vi "Untitled 4.vi"() -> ()   [LabVIEW 2016, in "Logger.syslog.lvclass"]
uses:
  Logger.syslog.lvclass
  <userlib>/_MGI/Error Reporter/MGI Error Reporter Dialog/MGI Error Reporter Dialog.lvclass
  C:/Program Files (x86)/National Instruments/LabVIEW 2016/user.lib/_MGI/Error Reporter/MGI Error Reporter Base/MGI Error Reporter Base.lvclass
  <userlib>/_OpenG.lib/numeric/numeric.llb/Random Number Within Range - DBL__ogtk.vi
  <userlib>/_MGI/Error Reporter/MGI Error Reporter Base/MGI Error Reporter Base.lvclass
panel:
  out "Already Running?":bool
  out "Error Log Directory Used":path
  in  "Log Error":bool
  in  "Stop":bool
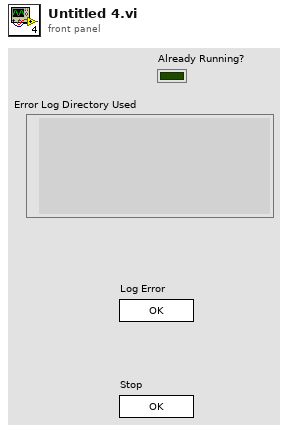
[diagram p1: front panel]
types:
  T1 = enum32{"Invalid", "Standard", "Closed", "Hidden", "Minimized", "Maximized"}
  T2 = enum32{"invalid app kind", "Development System", "Run Time System", "Student Edition", "Embedded LabVIEW", "Evaluation", "Custom"}
  T3 = cluster{"Core":cluster{"Current VI Reference":refnum<vi>, "Close Panel on Exit?":bool}, "Your Boolean data":bool, "Your string data":string}
  T4 = cluster{"Current VI Reference":refnum<vi>, "Close Panel on Exit?":bool}
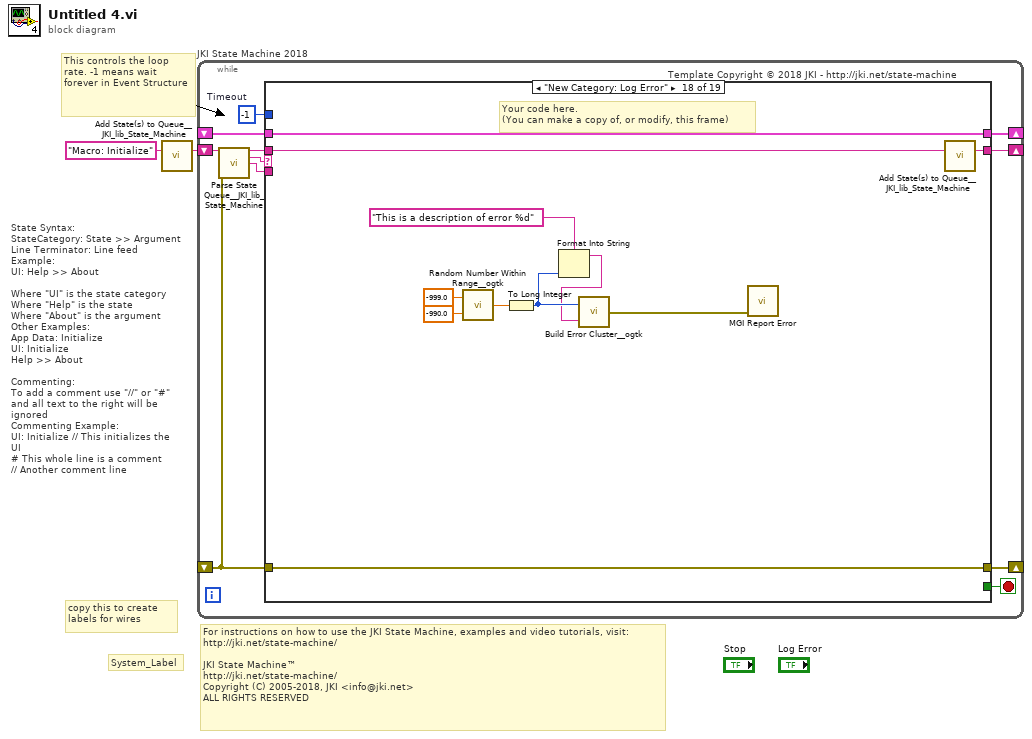
[diagram p0: block diagram]
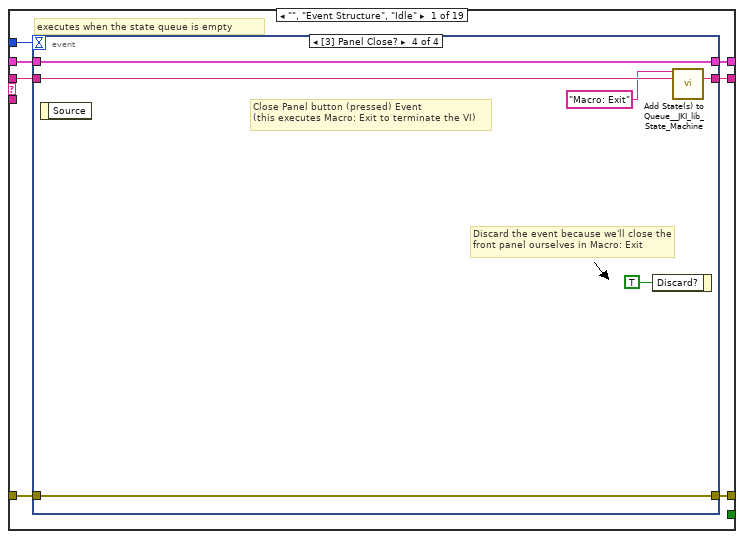
[diagram p2: hidden frame]
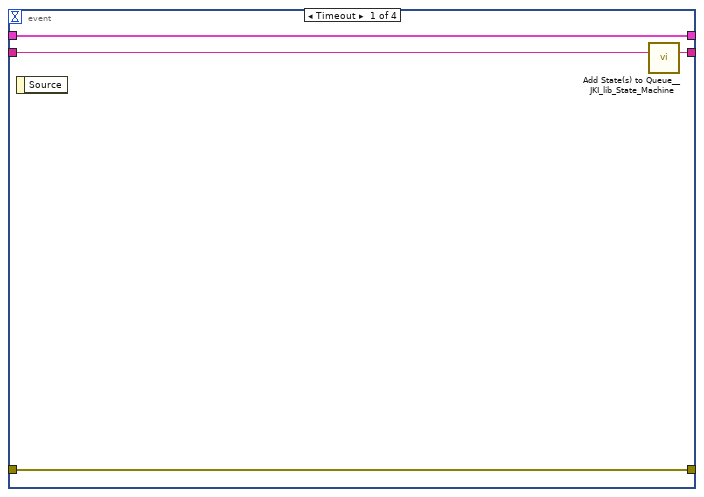
[diagram p3: hidden frame]
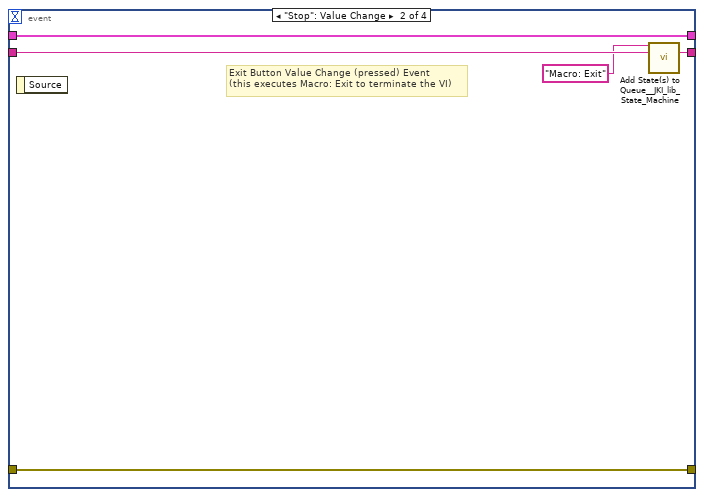
[diagram p4: hidden frame]
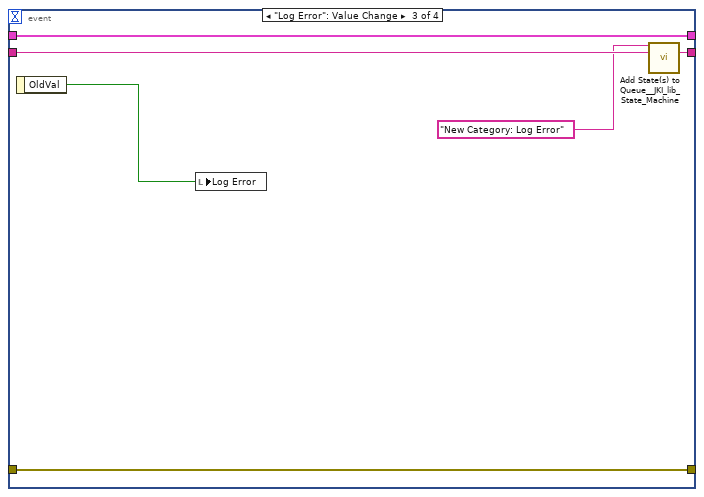
[diagram p5: hidden frame]
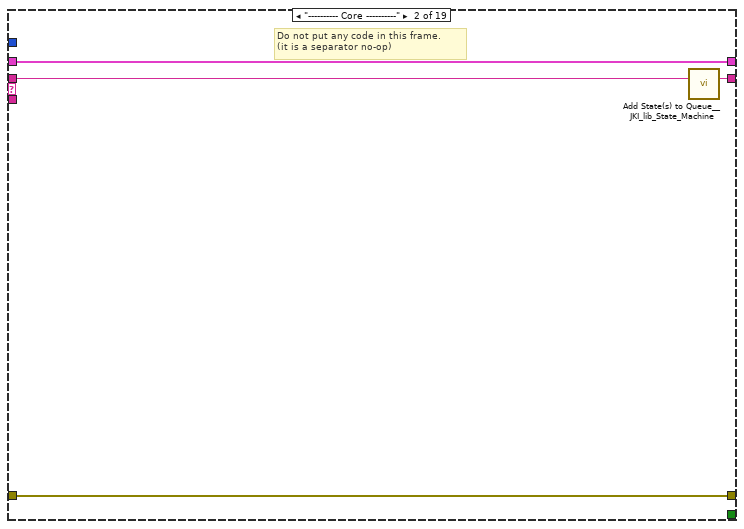
[diagram p6: hidden frame]
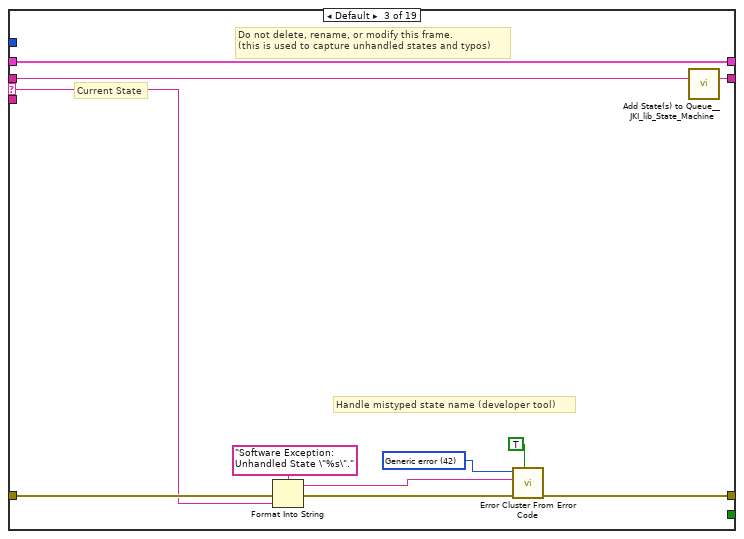
[diagram p7: hidden frame]
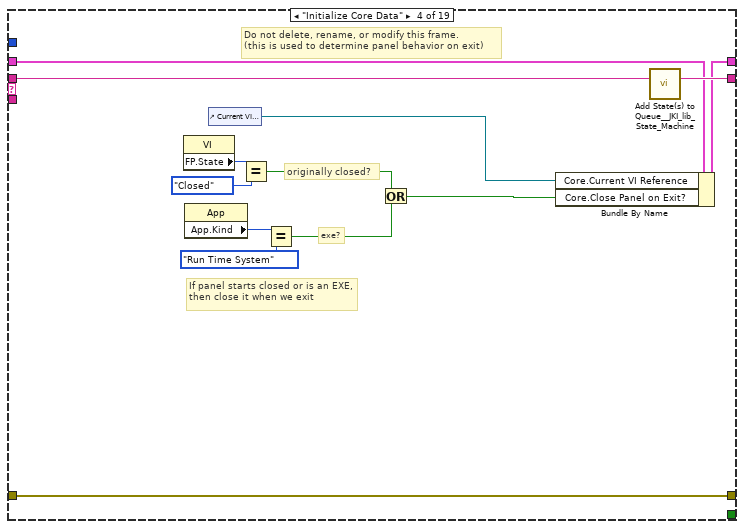
[diagram p8: hidden frame]
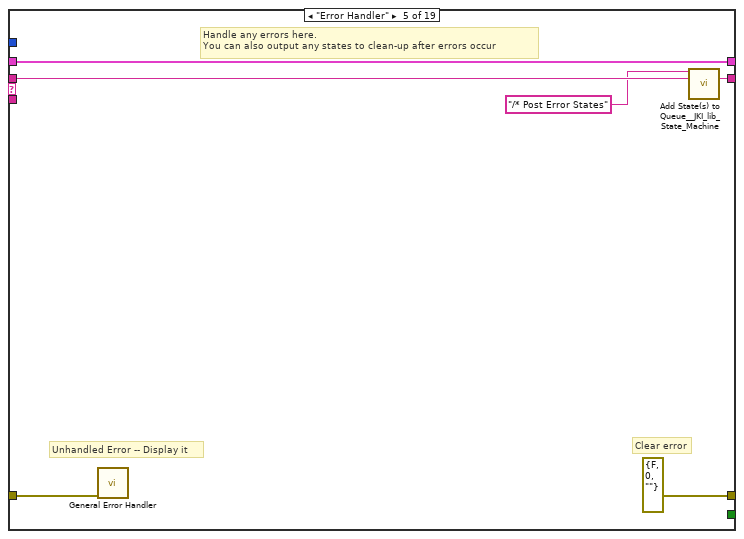
[diagram p9: hidden frame]
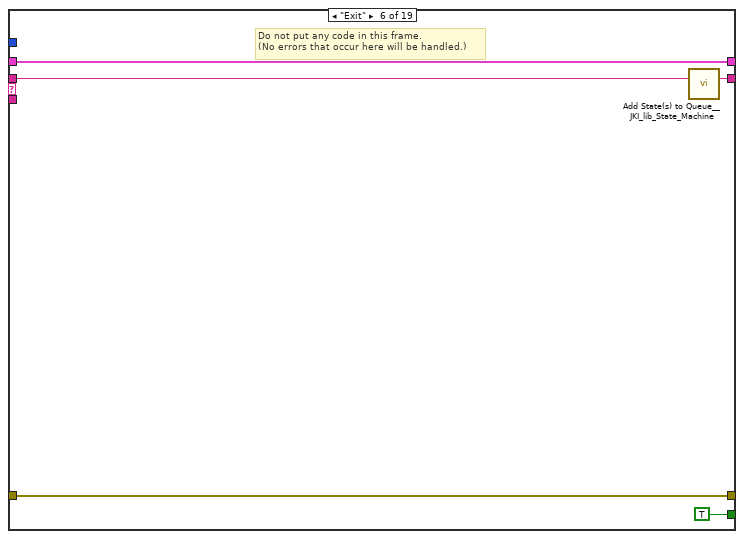
[diagram p10: hidden frame]
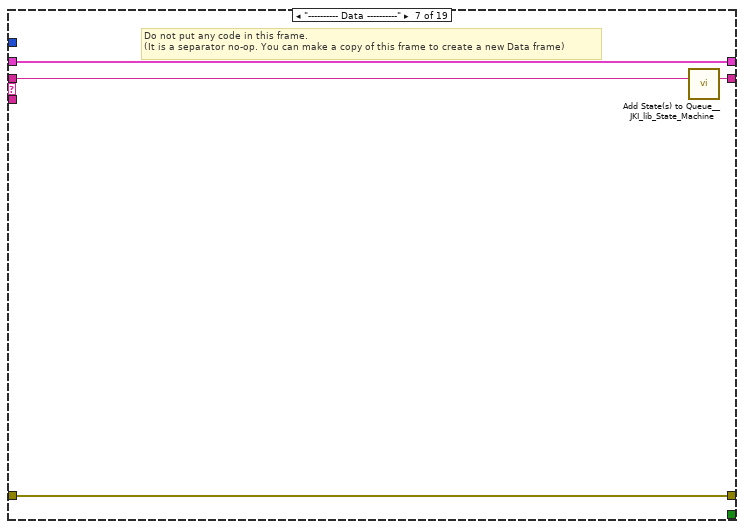
[diagram p11: hidden frame]
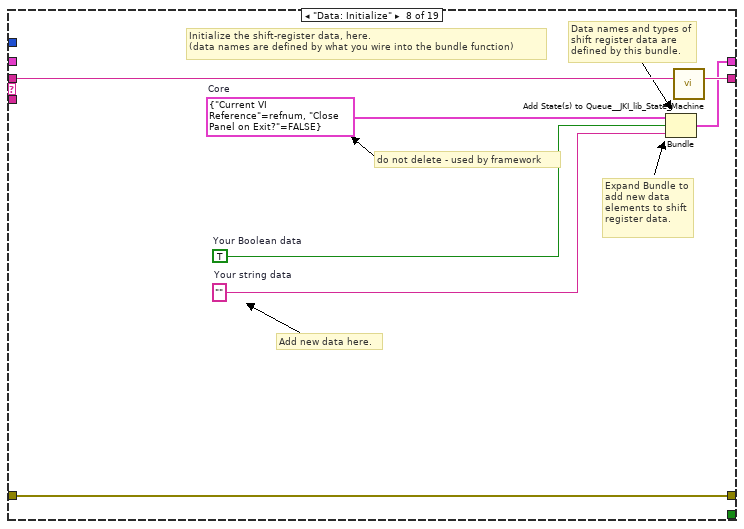
[diagram p12: hidden frame]
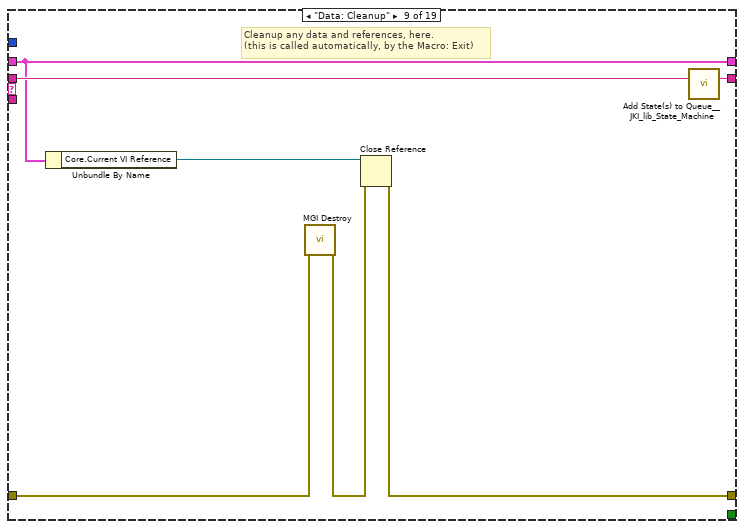
[diagram p13: hidden frame]
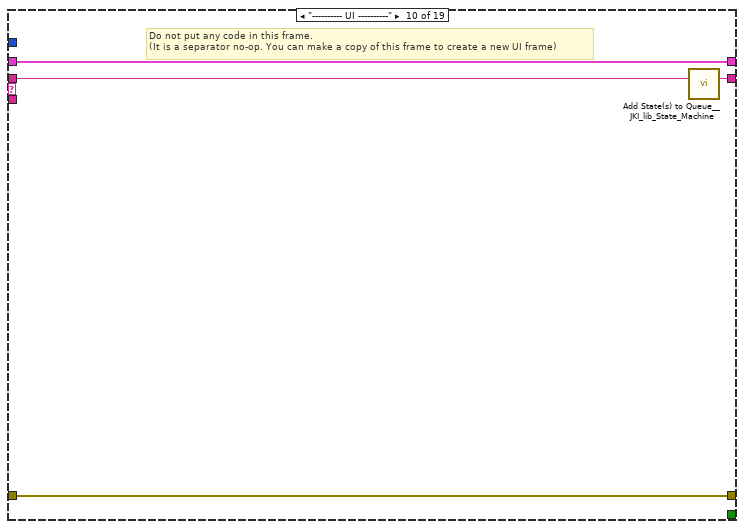
[diagram p14: hidden frame]
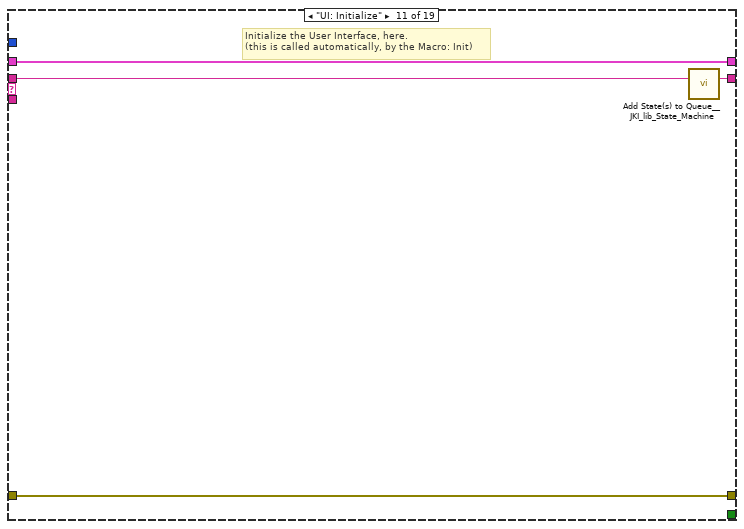
[diagram p15: hidden frame]
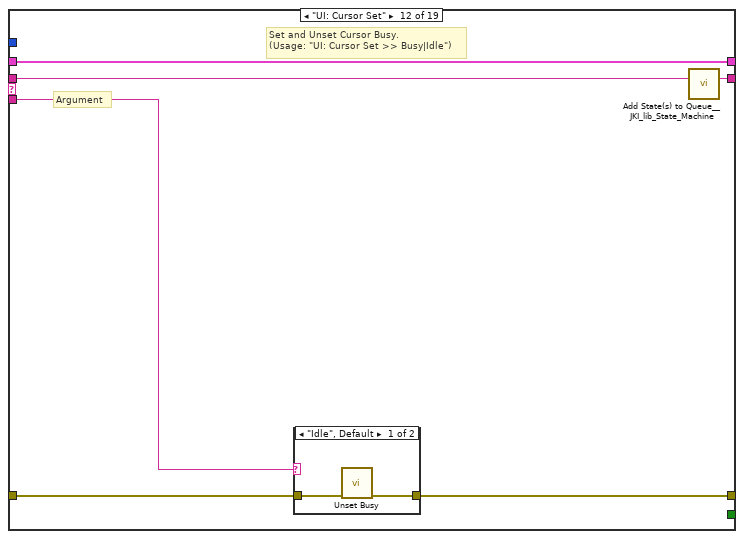
[diagram p16: hidden frame]
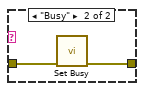
[diagram p17: hidden frame]
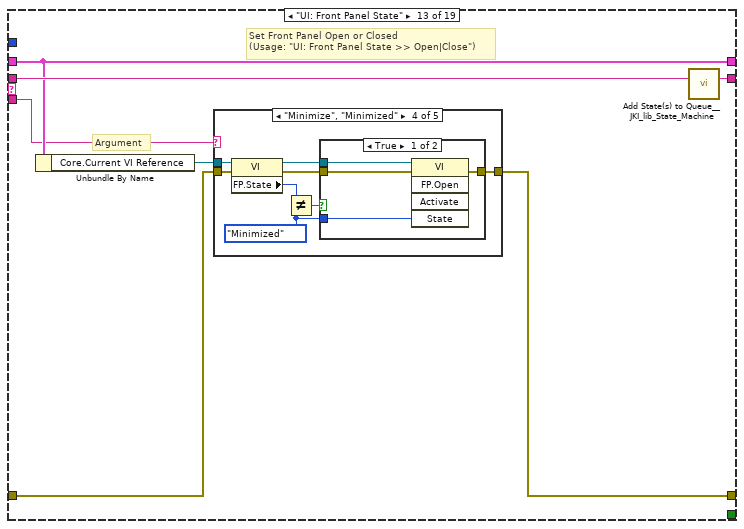
[diagram p18: hidden frame]
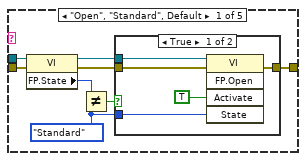
[diagram p19: hidden frame]
diagram:
  # "For instructions on how to use the JKI State Machine, examples and video tutorials, visit:\nhttp://jki.net/state-machine/\n\nJKI State Machine™\nhttp://jki.net/state-machine/\nCopyright (C) 2005-2018, JKI <info@jki.net>\nALL RIGHTS RESERVED"
  # "State Syntax:\nStateCategory: State >> Argument\nLine Terminator: Line feed\nExample:\nUI: Help >> About\n\nWhere \"UI\" is the state category\nWhere \"Help\" is the state\nWhere \"About\" is the argument\nOther Examples:\nApp Data: Initialize\nUI: Initialize\nHelp >> About\n\nCommenting:\nTo add a comment use \"//\" or \"#\" and all text to the right will be ignored\nCommenting Example:\nUI: Initialize // This initializes the UI\n# This whole line is a comment\n// Another comment line"
  # "copy this to create labels for wires"
  # "This controls the loop rate. -1 means wait forever in Event Structure"
  # "System_Label"
  n1 = call <vilib>:"Add State(s) to Queue__JKI_lib_State_Machine.vi"("State(s) in (\"\")"="Macro: Initialize") -> ("States Out"=w2:string)  [unwired: 14 in]
  n2 = while "JKI State Machine 2018" {
    shift-right: [w6] -> _
    shift-left: _ -> [w5]
    shift-right: [w9] -> _
    shift-left: _ -> [w3]
    shift-right: [w8] -> _
    shift-left: w2 -> [w10]
    stop <- w7 stop-if-true
    w4 = -1  # Timeout
    # "Template Copyright © 2018 JKI - http://jki.net/state-machine"
    n3 = call <vilib>:"Parse State Queue__JKI_lib_State_Machine.vi"("State Queue"=w10, "Error In (no error)"=w3) -> ("Remaining States"=w12:string, "Current State"=w13:string, "Arguments"=w11:string)  [unwired: 11 in]
    n4 = case shown="\"New Category: Log Error\"" w13 {
      selector: w13 -> [_ _ w46 _ _ _ _ _ _ _ _ _ _ _ _ _ _ _ _]
      tunnel: w12 -> [w20 w45 w50 w69 w75 w80 w84 w91 w98 w102 w106 w112 w123 w192 w197 w207 w211 w222 w240]
      tunnel: w11 -> [_ _ _ _ _ _ _ _ _ _ _ w107 w117 _ _ _ _ _ _]
      tunnel: w5 -> [w18 w42 w48 w62 w72 w78 w81 _ w94 w99 w104 w110 w119 w189 w194 w204 w208 w220 w238]
      tunnel: [w17 w43 w52 w66 errorcluster {"status"=FALSE, "code"=0, "source"=""} ("error out") w77 w82 w88 w95 w100 w103 w108 w120 w190 w195 w205 w209 w216 w235] -> w9
      tunnel: w3 -> [w16 w43 w51 w66 w71 w77 w82 w88 w93 w100 w103 w109 w121 w190 w195 w205 w209 w216 w236]
      tunnel: [w19 w44 w49 w68 w74 w79 w83 w90 w97 w101 w105 w111 w122 w191 w196 w206 w210 w221 w239] -> w8
      tunnel: [_ _ _ _ _ TRUE _ _ _ _ _ _ _ _ _ _ _ _ _] -> w7
      tunnel: [w15 w42 w48 w67 w72 w78 w81 w89 w94 w99 w104 w110 w119 w189 w194 w204 w208 w220 w238] -> w6
      tunnel: w4 -> [w14 _ _ _ _ _ _ _ _ _ _ _ _ _ _ _ _ _ _]
      frame "", "Event Structure", "Idle" {
        # "executes when the state queue is empty"
        n5 = event shown="[3] Panel Close?" {
          selector: _ -> [_ _ _ _]
          dyn-events: _ -> [_ _ _ _]
          timeout: w14 -> [_ _ _ _]
          tunnel: w20 -> [w24 w29 w35 w41]
          tunnel: [w23 w28 w34 w40] -> w19
          tunnel: w18 -> [w21 w26 w32 w38]
          tunnel: [w22 w27 w33 w39] -> w17
          tunnel: w16 -> [w22 w27 w33 w39]
          tunnel: [w21 w26 w32 w38] -> w15
          event Timeout {
            n6 = event-data() -> ()  [unwired: 1 in, 1 out]
            n7 = call <vilib>:"Add State(s) to Queue__JKI_lib_State_Machine.vi"("State(s) in (\"\")"=w24) -> ("States Out"=w23:string)  [unwired: 14 in]
          }
          event "Stop": Value Change {
            # "Exit Button Value Change (pressed) Event\n(this executes Macro: Exit to terminate the VI)"
            n8 = event-data() -> ()  [unwired: 1 in, 1 out]
            n9 = call <vilib>:"Add State(s) to Queue__JKI_lib_State_Machine.vi"("State(s) in Front (\"\")"="Macro: Exit", "State(s) in (\"\")"=w29) -> ("States Out"=w28:string)  [unwired: 13 in]
          }
          event "Log Error": Value Change {
            n10 = event-data() -> ("OldVal"=w30:bool)  [unwired: 1 in]
            n11 = local write "Log Error"(w30) -> ()
            n12 = call <vilib>:"Add State(s) to Queue__JKI_lib_State_Machine.vi"("State(s) in Front (\"\")"="New Category: Log Error", "State(s) in (\"\")"=w35) -> ("States Out"=w34:string)  [unwired: 13 in]
          }
          event Panel Close? {
            # "Discard the event because we'll close the front panel ourselves in Macro: Exit"
            # "Close Panel button (pressed) Event\n(this executes Macro: Exit to terminate the VI)"
            n13 = event-data() -> ()  [unwired: 1 in, 1 out]
            n14 = event-data("Discard?"=TRUE) -> ()  [unwired: 1 in, 1 out]
            n15 = call <vilib>:"Add State(s) to Queue__JKI_lib_State_Machine.vi"("State(s) in Front (\"\")"="Macro: Exit", "State(s) in (\"\")"=w41) -> ("States Out"=w40:string)  [unwired: 13 in]
          }
        }
      }
      frame "---------- Core ----------" {
        # "Do not put any code in this frame.\n(it is a separator no-op)"
        n16 = call <vilib>:"Add State(s) to Queue__JKI_lib_State_Machine.vi"("State(s) in (\"\")"=w45) -> ("States Out"=w44:string)  [unwired: 14 in]
      }
      frame Default {
        w55 = 42 items=["No error", "Argument error", "Memory is full", "Out of zone", "End of file", "File already open", "Generic file I/O error", "File not found", "File permission error", "Disk is full", "Duplicate path", "Too many files open", "System feature not enabled", "Resource file not found", "Cannot add resource", "Resource not found", "Image not found", "Image memory error", "Pen does not exist", "Config type invalid", "Config token not found", "Config parse error", "Config memory error", "Bad external code format", "Bad external code offset", "External code not present", "Null window", "Destroy window error", "Null menu", "Print aborted", "Bad print record", "Print driver error", "Windows error during printing", "Memory error during printing", "Print dialog error", "Generic print error", "Invalid device refnum", "Device not found", "Device parameter error", "Device unit error", "Cannot open device", "Device call aborted", "Generic error", "Cancelled by user", "Object ID too low", "Object ID too high", "Object not in heap", "Unknown heap", "Unknown object (invalid DefProc)", "Unknown object (DefProc not in table)", "Message out of range", "Invalid (null) method", "Unknown message", "Manager call not supported", "Bad address", "Network operation in progress", "Network operation timed out", "Connection is busy", "Network attribute not supported", "Network error", "Address in use", "System out of memory", "Connection aborted", "Connection refused", "Not connected", "Already connected", "Connection closed", "Initialization error (interapplication manager)", "Bad occurrence", "Wait on unbound occurrence handler", "Occurrence queue overflow", "Datalog type conflict", "Unused", "Unrecognized type (interapplication manager)", "Memory corrupt", "Failed to make temporary DLL", "Old CIN version", "Drag socket not found", "Failed to load drop-object", "Failed to register OLE object", "Failed to release OLE object", "Format specifier type mismatch", "Unknown format specifier", "Too few format specifiers", "Too many format specifiers", "Scan failed", "Newer CIN version", "Error converting to variant", "Runtime menu error", "Password tampered", "Variant attribute not found", "Incompatible variant data type", "Event data is not available", "Event Store is not present", "Occurrence is not found", "Event Queue is not created", "Event info is not available", "Refnum passed is NULL", "Error retrieving Class GUID", "Error retrieving CoClass GUID", "Error retrieving TypeLib GUID.", "Bad built application magic bytes.", "Specific driver is different from the specific driver associated with the Logical Name.", "There is no session opened to the class driver.", "Max Error", "MAX - Error with config objects", "MAX - Error loading configuration", "MAX - Group not supported"]
        # "Current State"
        # "Do not delete, rename, or modify this frame.\n(this is used to capture unhandled states and typos)"
        # "Handle mistyped state name (developer tool)"
        n17 = Format Into String(format string="Software Exception: Unhandled State \"%s\"." ("message"), error in=w51, w46) -> (resulting string=w54:string, error out=w53:errorcluster)  [unwired: 1 in]
        n18 = call <vilib>:"Error Cluster From Error Code.vi"("show call chain? (False)"=TRUE, "error in (no error)"=w53, "error message (\"\")"=w54, "error code (0)"=w55) -> ("error out"=w52:errorcluster)  [unwired: 5 in]
        n19 = call <vilib>:"Add State(s) to Queue__JKI_lib_State_Machine.vi"("State(s) in (\"\")"=w50) -> ("States Out"=w49:string)  [unwired: 14 in]
      }
      frame "Initialize Core Data" {
        # "Do not delete, rename, or modify this frame.\n(this is used to determine panel behavior on exit)"
        # "originally closed?"
        # "exe?"
        # "If panel starts closed or is an EXE, then close it when we exit"
        n20 = property class="VI"() -> ("FP.State"=w59:T1)  [unwired: 2 in, 2 out]
        n21 = property class="App"() -> ("App.Kind"=w65:T2)  [unwired: 2 in, 2 out]
        n22 = control-ref of="Current VI Reference"() -> (w60:refnum<vi>)
        n23 = Equal?(x=w59, y=T1."Closed" ("Front Panel Window:State")) -> (x = y?=w57:bool)
        n24 = Equal?(x=w65, y=T2."Run Time System" ("Application:Kind")) -> (x = y?=w63:bool)
        n25 = Or(x=w57, y=w63) -> (x .or. y?=w61:bool)
        n26 = Bundle By Name(cluster=w62, "Core.Current VI Reference"=w60, "Core.Close Panel on Exit?"=w61) -> (w67:T3)
        n27 = call <vilib>:"Add State(s) to Queue__JKI_lib_State_Machine.vi"("State(s) in (\"\")"=w69) -> ("States Out"=w68:string)  [unwired: 14 in]
      }
      frame "Error Handler" {
        # "Unhandled Error -- Display it"
        # "Handle any errors here.\nYou can also output any states to clean-up after errors occur"
        # "Clear error"
        n28 = call <vilib>:"General Error Handler.vi"("error in (no error)"=w71) -> ()  [unwired: 10 in, 5 out]
        n29 = call <vilib>:"Add State(s) to Queue__JKI_lib_State_Machine.vi"("State(s) in Front (\"\")"="/* Post Error States", "State(s) in (\"\")"=w75) -> ("States Out"=w74:string)  [unwired: 13 in]
      }
      frame "Exit" {
        # "Do not put any code in this frame.\n(No errors that occur here will be handled.)"
        n30 = call <vilib>:"Add State(s) to Queue__JKI_lib_State_Machine.vi"("State(s) in (\"\")"=w80) -> ("States Out"=w79:string)  [unwired: 14 in]
      }
      frame "---------- Data ----------" {
        # "Do not put any code in this frame.\n(It is a separator no-op. You can make a copy of this frame to create a new Data frame)"
        n31 = call <vilib>:"Add State(s) to Queue__JKI_lib_State_Machine.vi"("State(s) in (\"\")"=w84) -> ("States Out"=w83:string)  [unwired: 14 in]
      }
      frame "Data: Initialize" {
        w85 = T4 {"Current VI Reference"=refnum, "Close Panel on Exit?"=FALSE}  # Core
        w87 = TRUE  # Your Boolean data
        w86 = ""  # Your string data
        # "do not delete - used by framework"
        # "Expand Bundle to add new data elements to shift register data."
        # "Add new data here."
        # "Data names and types of shift register data are defined by this bundle."
        # "Initialize the shift-register data, here.\n(data names are defined by what you wire into the bundle function)"
        n32 = Bundle("Core"=w85, "Your Boolean data"=w87, "Your string data"=w86) -> (w89:T3)  [unwired: 1 in]
        n33 = call <vilib>:"Add State(s) to Queue__JKI_lib_State_Machine.vi"("State(s) in (\"\")"=w91) -> ("States Out"=w90:string)  [unwired: 14 in]
      }
      frame "Data: Cleanup" {
        # "Cleanup any data and references, here.\n(this is called automatically, by the Macro: Exit)"
        n34 = Unbundle By Name(w94) -> ("Core.Current VI Reference"=w96:refnum<vi>)
        n35 = call <userlib>:"MGI Destroy.vi"("error in (no error)"=w93) -> ("error out"=w92:errorcluster)  [unwired: 10 in]
        n36 = Close Reference(reference=w96, error in (no error)=w92) -> (error out=w95:errorcluster)
        n37 = call <vilib>:"Add State(s) to Queue__JKI_lib_State_Machine.vi"("State(s) in (\"\")"=w98) -> ("States Out"=w97:string)  [unwired: 14 in]
      }
      frame "---------- UI ----------" {
        # "Do not put any code in this frame.\n(It is a separator no-op. You can make a copy of this frame to create a new UI frame)"
        n38 = call <vilib>:"Add State(s) to Queue__JKI_lib_State_Machine.vi"("State(s) in (\"\")"=w102) -> ("States Out"=w101:string)  [unwired: 14 in]
      }
      frame "UI: Initialize" {
        # "Initialize the User Interface, here.\n(this is called automatically, by the Macro: Init)"
        n39 = call <vilib>:"Add State(s) to Queue__JKI_lib_State_Machine.vi"("State(s) in (\"\")"=w106) -> ("States Out"=w105:string)  [unwired: 14 in]
      }
      frame "UI: Cursor Set" {
        # "Argument"
        # "Set and Unset Cursor Busy.\n(Usage: \"UI: Cursor Set >> Busy|Idle\")"
        n40 = case shown="\"Idle\", Default" w107 {
          tunnel: w109 -> [w114 w116]
          tunnel: [w113 w115] -> w108
          frame "Idle", Default {
            n41 = call <vilib>:"Unset Busy.vi"("error in (no error)"=w114) -> ("error out"=w113:errorcluster)  [unwired: 10 in]
          }
          frame "Busy" {
            n42 = call <vilib>:"Set Busy.vi"("error in (no error)"=w116) -> ("error out"=w115:errorcluster)  [unwired: 9 in, 1 out]
          }
        }
        n43 = call <vilib>:"Add State(s) to Queue__JKI_lib_State_Machine.vi"("State(s) in (\"\")"=w112) -> ("States Out"=w111:string)  [unwired: 14 in]
      }
      frame "UI: Front Panel State" {
        # "Argument"
        # "Set Front Panel Open or Closed\n(Usage: \"UI: Front Panel State >> Open|Close\")"
        n44 = Unbundle By Name(w119) -> ("Core.Current VI Reference"=w118:refnum<vi>)
        n45 = case shown="\"Minimize\", \"Minimized\"" w117 {
          tunnel: w121 -> [w129 w144 w155 w168 w181]
          tunnel: [w131 w145 w157 w170 w183] -> w120
          tunnel: w118 -> [w130 w142 w156 w169 w182]
          frame "Open", "Standard", Default {
            w124 = T1."Standard" ("State")
            n46 = property class="VI"(reference=w130, error in=w129) -> (reference out=w127:refnum<vi>, error out=w128:errorcluster, "FP.State"=w126:T1)
            n47 = Not Equal?(x=w126, y=w124) -> (x != y?=w125:bool)
            n48 = case shown="True" w125 {
              tunnel: [w135 w137] -> w131
              tunnel: w128 -> [w134 w137]
              tunnel: w127 -> [w133 _]
              tunnel: w124 -> [w132 _]
              frame True {
                n49 = invoke class="VI" method="FP.Open"(reference=w133, error in=w134, "Activate"=TRUE, "State"=w132) -> (error out=w135:errorcluster)  [unwired: 1 in, 4 out]
              }
              frame False {
              }
            }
          }
          frame "Close", "Closed" {
            n50 = property class="VI"(reference=w142, error in=w144) -> (reference out=w141:refnum<vi>, error out=w143:errorcluster, "FP.State"=w139:T1)
            n51 = Not Equal?(x=w139, y=T1."Closed" ("Front Panel Window:State")) -> (x != y?=w138:bool)
            n52 = case shown="True" w138 {
              tunnel: [w146 w149] -> w145
              tunnel: w143 -> [w146 w148]
              tunnel: w141 -> [_ w147]
              frame False {
              }
              frame True {
                n53 = invoke class="VI" method="FP.Close"(reference=w147, error in=w148) -> (error out=w149:errorcluster)  [unwired: 1 in, 2 out]
              }
            }
          }
          frame "Hidden", "Hide" {
            w150 = T1."Hidden" ("State")
            n54 = property class="VI"(reference=w156, error in=w155) -> (reference out=w153:refnum<vi>, error out=w154:errorcluster, "FP.State"=w152:T1)
            n55 = Not Equal?(x=w152, y=w150) -> (x != y?=w151:bool)
            n56 = case shown="True" w151 {
              tunnel: [w161 w162] -> w157
              tunnel: w154 -> [w160 w162]
              tunnel: w153 -> [w159 _]
              tunnel: w150 -> [w158 _]
              frame True {
                n57 = invoke class="VI" method="FP.Open"(reference=w159, error in=w160, "State"=w158) -> (error out=w161:errorcluster)  [unwired: 2 in, 4 out]
              }
              frame False {
              }
            }
          }
          frame "Minimize", "Minimized" {
            w163 = T1."Minimized" ("State")
            n58 = property class="VI"(reference=w169, error in=w168) -> (reference out=w166:refnum<vi>, error out=w167:errorcluster, "FP.State"=w165:T1)
            n59 = Not Equal?(x=w165, y=w163) -> (x != y?=w164:bool)
            n60 = case shown="True" w164 {
              tunnel: [w174 w175] -> w170
              tunnel: w167 -> [w173 w175]
              tunnel: w166 -> [w172 _]
              tunnel: w163 -> [w171 _]
              frame True {
                n61 = invoke class="VI" method="FP.Open"(reference=w172, error in=w173, "State"=w171) -> (error out=w174:errorcluster)  [unwired: 2 in, 4 out]
              }
              frame False {
              }
            }
          }
          frame "Maximize", "Maximized" {
            w176 = T1."Maximized" ("State")
            n62 = property class="VI"(reference=w182, error in=w181) -> (reference out=w179:refnum<vi>, error out=w180:errorcluster, "FP.State"=w178:T1)
            n63 = Not Equal?(x=w178, y=w176) -> (x != y?=w177:bool)
            n64 = case shown="True" w177 {
              tunnel: [w187 w188] -> w183
              tunnel: w180 -> [w186 w188]
              tunnel: w179 -> [w185 _]
              tunnel: w176 -> [w184 _]
              frame True {
                n65 = invoke class="VI" method="FP.Open"(reference=w185, error in=w186, "State"=w184) -> (error out=w187:errorcluster)  [unwired: 2 in, 4 out]
              }
              frame False {
              }
            }
          }
        }
        n66 = call <vilib>:"Add State(s) to Queue__JKI_lib_State_Machine.vi"("State(s) in (\"\")"=w123) -> ("States Out"=w122:string)  [unwired: 14 in]
      }
      frame "---------- Macro ----------" {
        # "Do not put any code in this frame.\n(It is a separator no-op. You can make a copy of this frame to create a new Macro frame)"
        n67 = call <vilib>:"Add State(s) to Queue__JKI_lib_State_Machine.vi"("State(s) in (\"\")"=w192) -> ("States Out"=w191:string)  [unwired: 14 in]
      }
      frame "Macro: Initialize" {
        w193 = "Data: Initialize\nInitialize Core Data\nUI: Initialize\nUI: Front Panel State >> Open\nNew Category: Start Error Logger"  # Data: Initialize Initialize Core Data UI: Initialize UI: Front Panel State >> Open New Category: Start Error Logger
        # "Initialization Macro\n(This is called once, when the VI starts)"
        n68 = call <vilib>:"Add State(s) to Queue__JKI_lib_State_Machine.vi"("State(s) in Front (\"\")"=w193, "State(s) in (\"\")"=w197) -> ("States Out"=w196:string)  [unwired: 13 in]
      }
      frame "Macro: Exit" {
        # "Exit Macro\n(This is called once, when the VI exits)"
        n69 = Unbundle By Name(w204) -> ("Core.Close Panel on Exit?"=w203:bool)
        n70 = Select(t="UI: Front Panel State >> Close", s=w203, f="") -> (s? t:f=w200:string)
        n71 = call <vilib>:"Add State(s) to Queue__JKI_lib_State_Machine.vi"("State(s) in (\"\")"=w200, "State(s) at Back (\"\")"="Data: Cleanup\nExit") -> ("States Out"=w198:string)  [unwired: 13 in]
        n72 = call <vilib>:"Add State(s) to Queue__JKI_lib_State_Machine.vi"("State(s) in Front (\"\")"=w198, "State(s) in (\"\")"=w207) -> ("States Out"=w206:string)  [unwired: 13 in]
      }
      frame "---------- New Category ----------" {
        # "Template Separator\n(You can make a copy of, or modify, this frame)"
        n73 = call <vilib>:"Add State(s) to Queue__JKI_lib_State_Machine.vi"("State(s) in (\"\")"=w211) -> ("States Out"=w210:string)  [unwired: 14 in]
      }
      frame "New Category: Log Error" {
        # "Your code here.\n(You can make a copy of, or modify, this frame)"
        n74 = call-poly <userlib>:"Random Number Within Range__ogtk.vi"("High"=-999.0, "Low"=-990.0) -> ("Random Number"=w219:dbl)  [unwired: 3 in]
        n75 = To Long Integer(number=w219) -> (32bit integer=w214:i32)
        n76 = Format Into String(format string="This is a description of error %d" ("String to Prepend to source (\"\")"), w214) -> (resulting string=w212:string)  [unwired: 2 in, 1 out]
        n77 = call <userlib>:"Build Error Cluster__ogtk.vi"("String to Prepend to source (\"\")"=w212, "code"=w214) -> ("error out"=w215:errorcluster)
        n78 = call <userlib>:"MGI Report Error.vi"("error in"=w215) -> ()  [unwired: 10 in, 1 out]
        n79 = call <vilib>:"Add State(s) to Queue__JKI_lib_State_Machine.vi"("State(s) in (\"\")"=w222) -> ("States Out"=w221:string)  [unwired: 14 in]
      }
      frame "New Category: Start Error Logger" {
        # "Your code here.\n(You can make a copy of, or modify, this frame)"
        n80 = call-dynamic "MGI Set Custom Error Codes.vi"("Custom Name[i] (Default Set)"=string[] ["error 1", "error 2", "error 3"], "Custom Code[i] (Default Set)"=i32[] [-999, -998, -997], "MGI Error Reporter Base In"=refnum<class "MGI Error Reporter Dialog.lvclass"> refnum ("Reporter Dialog.lvclass")) -> ("MGI Error Reporter Base Out"=w227:refnum<class "MGI Error Reporter Dialog.lvclass">)  [unwired: 8 in]
        n81 = call <userlib>:"MGI Set Logging Parameters.vi"("Max # Log Files (Don't change)"=-2, "Max # Errors to Log (Don't change)"=-2, "MGI Error Reporter Base In"=w227) -> ("MGI Error Reporter Base Out"=w226:refnum<class "MGI Error Reporter Dialog.lvclass">)  [unwired: 8 in]
        n82 = call <userlib>:"Create Dir if Non-Existant__ogtk.vi"("error in (no error)"=w236, "Directory Path"=path "C:/Users/Patrick/Desktop/Error Log" ("Error Log Directory \n(Not a Path: Shared Docs\\Caller Prefix)\n(\"\" Path: Turn off logging)")) -> ("error out"=w234:errorcluster, "dup Directory Path"=w233:path)  [unwired: 7 in, 1 out]
        n83 = call <userlib>:"MGI Create.vi"("error in (no error)"=w234, "Error Log Directory \n(Not a Path: Shared Docs\\Caller Prefix)\n(\"\" Path: Turn off logging)"=w233, "Reporter Dialog.lvclass"=w226) -> ("error out"=w231:errorcluster, "Error Log Directory Used"=→"Error Log Directory Used":path, "Already Running?"=→"Already Running?":bool)  [unwired: 6 in]
        n84 = call <userlib>:"MGI Show UI.vi"("error in (no error)"=w231) -> ("error out"=w235:errorcluster)  [unwired: 10 in]
        n85 = call <vilib>:"Add State(s) to Queue__JKI_lib_State_Machine.vi"("State(s) in (\"\")"=w240) -> ("States Out"=w239:string)  [unwired: 14 in]
      }
    }
  }
